vi "UTIL Probe Reference.vi"(8 "error in (no error)":errorcluster, 11 "niDTS Comm Telnet in":refnum<class "niDTS Comm Telnet.lvclass">) -> (0 "error out":errorcluster, 2 "VI Refnum":refnum<vi>, 3 "niDTS Comm Telnet out":refnum<class "niDTS Comm Telnet.lvclass">)   [LabVIEW 2015, in "niDTS CommLib.lvlib" / "niDTS Comm Telnet.lvclass"]
uses:
  niDTS Comm Telnet.lvclass
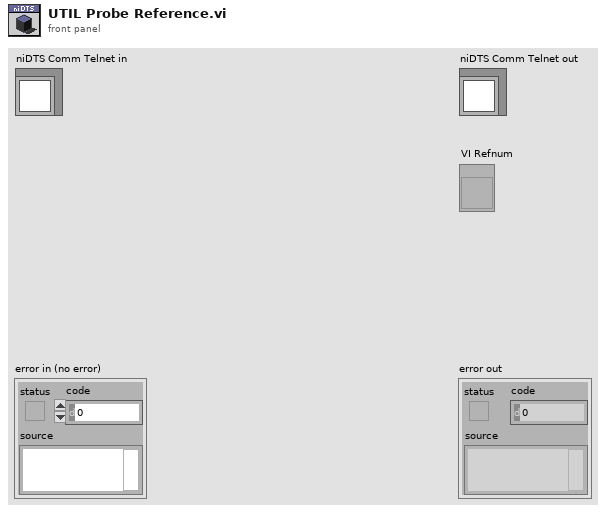
[diagram p1: front panel]
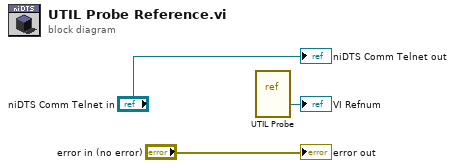
[diagram p0: block diagram]
diagram:
  n1 = vi-ref "UTIL Probe.vi"() -> (→"VI Refnum":refnum<vi>)
  "error out" <- "error in (no error)"
  "niDTS Comm Telnet out" <- "niDTS Comm Telnet in"
